vi "Funktionen Schalten Compact LP.vi"(8 "Fehler (Eingang)":errorcluster) -> (0 "Fehler (Ausgang)":errorcluster, 2 "Zustand":T1)   [LabVIEW 2020, in "Allgemein.lvlib"]
uses:
  Allgemein.lvlib
  Funktionstasten/Zustaende.ctl
  FGV Zustaende Aktionen.ctl
  Verwaltung/FGV OUT Aktionen.ctl
  Regler/FGV Daten Regler Aktionen.ctl
  Aktion FGV Messbetrieb.ctl
  Aktionen FGV Dichtheitstest.ctl
  Verwaltung/Verwaltung - cRIO.lvlib
  Regler/Regler.lvlib
  Funktionstasten/Funktionstasten.lvlib
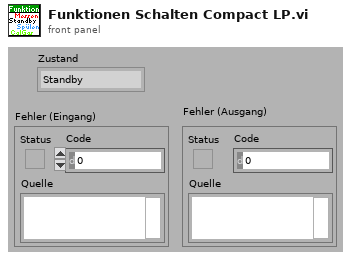
[diagram p1: front panel]
types:
  T1 = typedef "Funktionstasten.lvlib/Zustaende.ctl" = enum16{"Standby", "Pause", "Eco", "Messen", "Kalibrieren", "Spülen Filter", "Spülen Leitung", "Umgebungsluft", "0-Gas", "Cal-Gas", "CG zu PNS", "-------------", "Init 1", "Init 2", "Init 3", "Init 4", "Messen vorbereiten", "Messen durchführen", "Exit"}
  T2 = typedef "Allgemein.lvlib/Aktion FGV Messbetrieb.ctl" = enum16{"lesen", "schreiben"}
  T3 = typedef "Regler.lvlib/FGV Daten Regler Aktionen.ctl" = enum16{"lesen", "Out%", "Heizung EIN"}
  T4 = typedef "Verwaltung - cRIO.lvlib/FGV OUT Aktionen.ctl" = enum16{"lesen", "ANA OUT", "DO 0-31", "DO 32-47"}
  T5 = typedef "Allgemein.lvlib/FGV Zustaende Aktionen.ctl" = enum16{"lesen", "Zustand PC", "Zustand cRIO", "Bildnummer", "Samplepoint", "Sysloglevel"}
  T6 = typedef "Allgemein.lvlib/Aktionen FGV Dichtheitstest.ctl" = enum16{"lesen", "schreiben"}
  T7 = typedef "EPA 1065.lvlib/Dichtheitstest 1065-345.lvlib/Aktion Leak check durchfuehren.ctl" = enum16{"initialisieren", "Unterdruck erzeugen", "Ventile schließen", "Warten", "Auswertung", "fertig", "PDF erstellen", "abbrechen"}
  T8 = typedef "Erweiterte Konfig.lvlib/Aktionen Dichtheitstest.ctl" = enum16{"Initialisieren", "Unterdruck aufbauen", "Prop schließen", "Warten", "Auswertung", "Fertig"}
  T9 = cluster{"-23Y1":bool, "-23Y2":bool, "-23Y3":bool, "-23Y4":bool, "-23Y5":bool, "-27Y2":bool, "-20Y5":bool, "-20Y6":bool, "-20Y7":bool, "-20Y8":bool, "-27Y3":bool, "-27Y4":bool, "Pumpe":bool, "Kondensat":bool, "-22Y3":bool, "-20Y2":bool, "-21Y3":bool, "Absaugung":bool, "-21Y5":bool, "CG zu Entnahme":bool}
  T10 = cluster{"-23Y1 (Reserve)":bool, "-23Y2 (Reserve)":bool, "-23Y3 (CG1-8)":bool, "-23Y4 (N2)":bool, "-23Y5":bool, "-27Y2":bool, "-20Y5":bool, "-20Y6":bool, "-20Y7":bool, "-20Y8":bool, "-27Y3":bool, "-27Y4":bool, "Pumpe":bool, "Kondensat":bool, "-22Y3":bool, "-20Y2":bool, "-21Y3":bool, "Absaugung":bool, "-21Y5":bool, "CG zu Entnahme":bool, "-20Y2 (CG1)":bool, "-20Y3 (CG2)":bool, "-20Y4 (CG3)":bool, "-20Y5 (CG4)":bool, "-20Y6 (CG5)":bool, "-20Y7 (CG6)":bool, "-20Y8 (CG7)":bool, "-21Y1 (CG8)":bool}
  T11 = typedef "Verwaltung - cRIO.lvlib/Digital Ausgaenge 32-63.ctl" = cluster{"O32: Messgaspumpe EIN":bool, "O33: (Umgebungsluftpumpe)":bool, "O34: (Kondensatpumpe GK)":bool, "O35: Klima/Lüfter EIN":bool, "O36: Versorgung Heizungen":bool, "O37: Versorgung Heizungen":bool, "O38: (Gaskühler EIN (Freigabe))":bool, "O39: Störung FAS LP":bool, "O40: (Heizung Filterblock)":bool, "O41: Heizung HL zu FT-IR":bool, "O42: Heizung HL Extern SP1":bool, "O43: Heizung HL Extern SP2":bool, "O44: Heizung Reserve":bool, "O45: Heizung Reserve":bool, "O46: Statusbeleuchtung grün":bool, "O47: Statusbeleuchtung rot":bool}
  T12 = typedef "Verwaltung - cRIO.lvlib/Digital Ausgaenge 0-31.ctl" = cluster{"O0: Druckluft Versorgung":bool, "O1: CG 1 (FB Eingang 1)":bool, "O2: CG 2 (Kühlung FT-IR EIN)":bool, "O3: CG 3 (FB Bypass)":bool, "O4: CG 4 (FB CalGas)":bool, "O5: CG 5 (FB spülen/UL)":bool, "O6: CG 6 (FB zum FT-IR)":bool, "O7: CG 7 (FB zum FID)":bool, "O8: CG 8 (FB Reserve)":bool, "O9: (FB Reserve)":bool, "O10: (FB Umgebungsluft FID)":bool, "O11: (FB zum Gaskühler)":bool, "O12: FB Stickstoff zu FT-IR":bool, "O13: Optikbox FT-IR spülen":bool, "O14: (Purifier deaktivieren)":bool, "O15: (Umschaltung Purifier/Stickstoff)":bool, "O16: N2 Einblasung":bool, "O17: LSP LN2 Nachfüllung":bool, "O18: (Reserve)":bool, "O19: (Pumpe Eingang1)":bool, "O20: (Pumpe Eingang2)":bool, "O21: (Pumpe Spülen1)":bool, "O22: (Pumpe Spülen2)":bool, "O23: (Reserve)":bool, "O24: CalGas 1":bool, "O25: CalGas 2":bool, "O26: CG 3-8 (CalGas 3)":bool, "O27: Stickstoff aufschalten":bool, "O28: CG zu PNS":bool, "O29: FTIR Standby Spülung":bool, "O30: CG zu Entnahme(T90)":bool, "O31: (Purifier regenerieren)":bool}
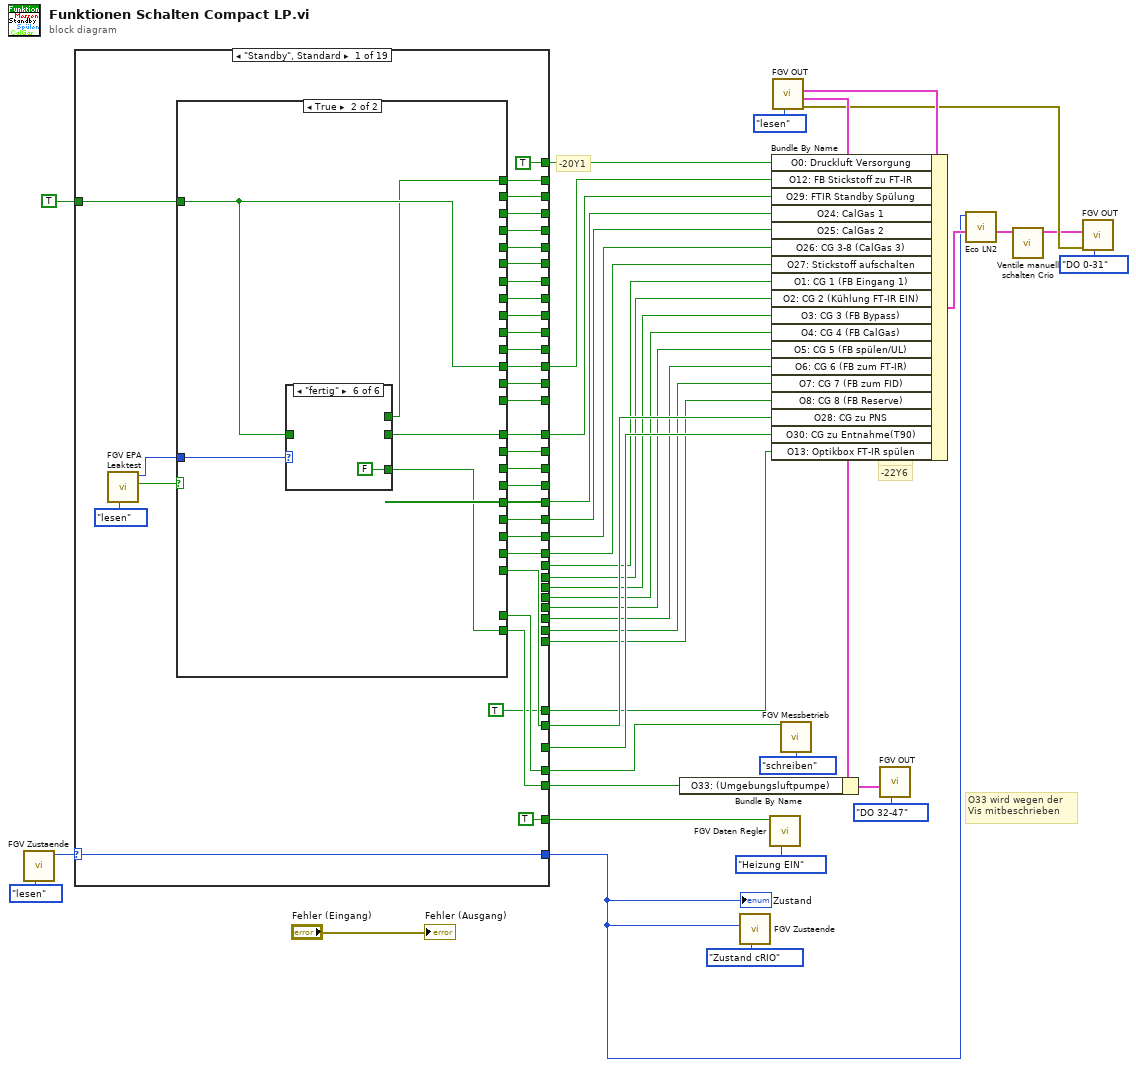
[diagram p0: block diagram]
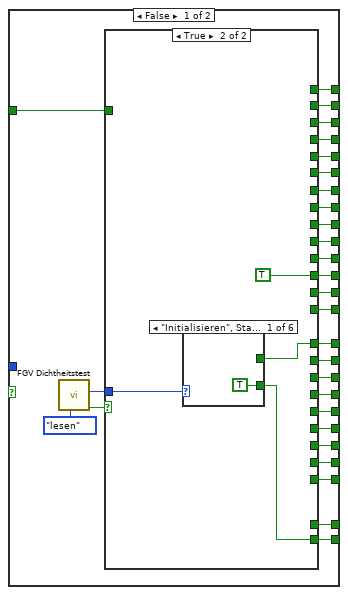
[diagram p2: hidden frame]
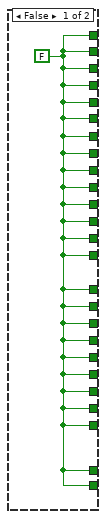
[diagram p3: hidden frame]
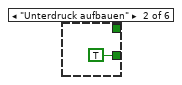
[diagram p4: hidden frame]
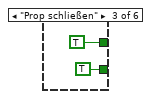
[diagram p5: hidden frame]
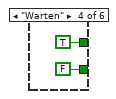
[diagram p6: hidden frame]
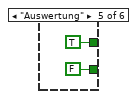
[diagram p7: hidden frame]
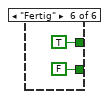
[diagram p8: hidden frame]
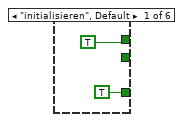
[diagram p9: hidden frame]
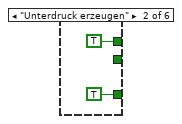
[diagram p10: hidden frame]
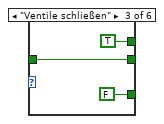
[diagram p11: hidden frame]
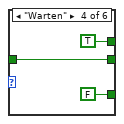
[diagram p12: hidden frame]
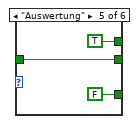
[diagram p13: hidden frame]
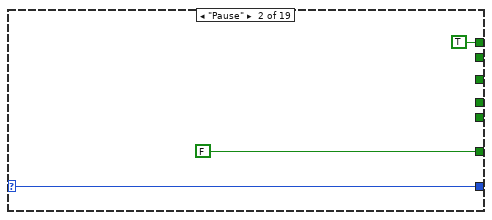
[diagram p14: hidden frame]
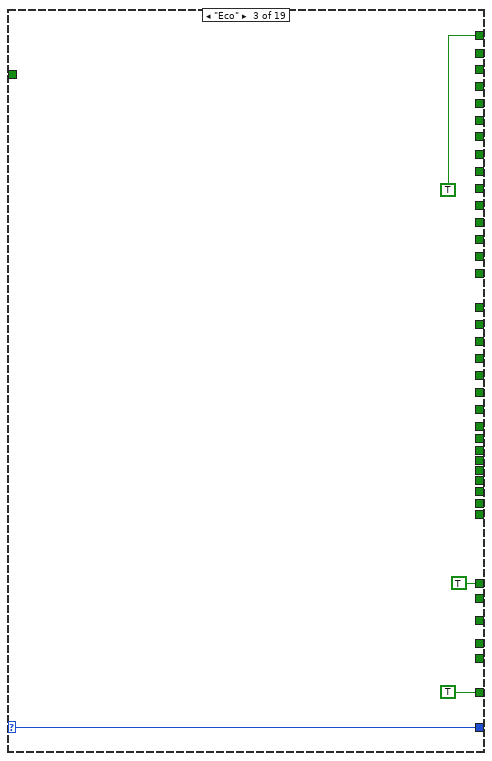
[diagram p15: hidden frame]
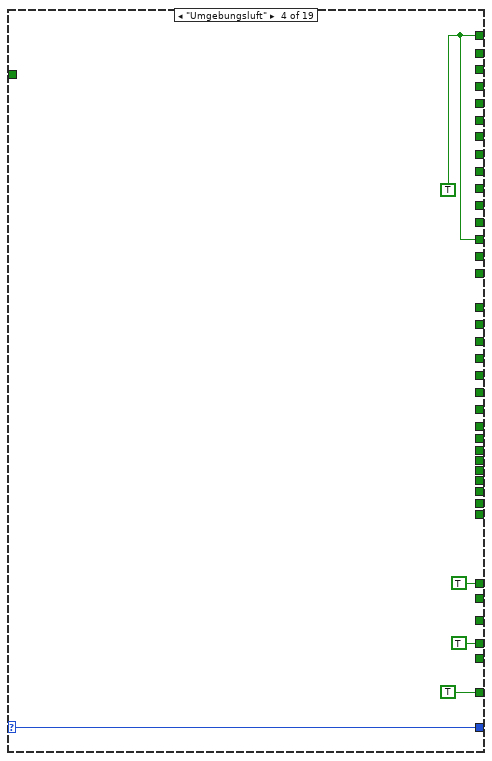
[diagram p16: hidden frame]
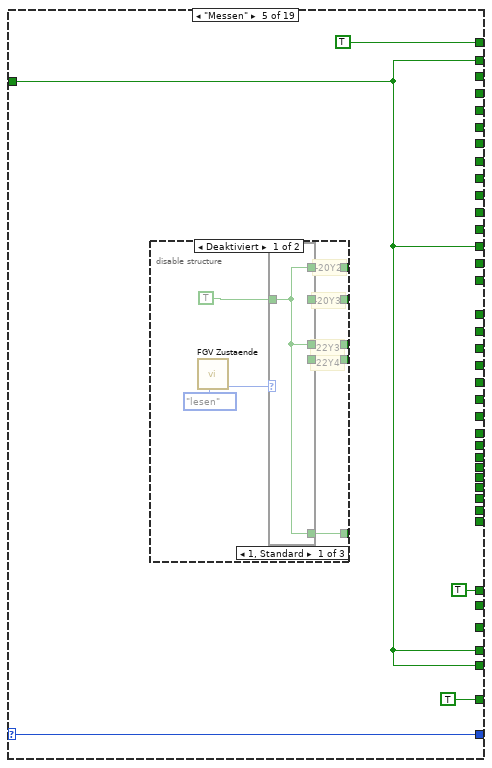
[diagram p17: hidden frame]
diagram:
  # "O33 wird wegen der \nVis mitbeschrieben"
  # "-20Y1"
  # "-22Y6"
  # "-22Y5"
  # "-22Y4"
  n1 = call "FGV Zustaende.vi"("Aktionen"=FGV_Zustaende_Aktionen."lesen") -> ("Zustand PC"=w31:T1)  [unwired: 6 in, 4 out]
  n2 = case shown="\"Standby\", Standard" w31 {
    selector: w31 -> [w72 w138 w142 w147 w152 w195 w219 w224 w241 w268 w331 _ _ _ _ _ w379 w381 _]
    tunnel: [w72 w138 w142 w147 w152 w195 w219 w224 w241 w268 w331 _ _ _ _ _ w379 w381 _] -> w14
    tunnel: [w70 _ _ _ w149 w189 _ w221 _ w265 w328 _ _ _ _ _ _ _ _] -> _
    tunnel: [w69 _ _ _ _ w188 _ _ _ _ _ _ _ _ _ _ _ _ _] -> _
    tunnel: [w67 _ _ _ _ w186 _ _ w238 w264 w327 _ _ _ _ _ _ _ _] -> _
    tunnel: [w66 _ _ _ _ w185 _ _ _ w263 w326 _ _ _ _ _ _ _ _] -> _
    tunnel: [w65 _ _ _ _ w184 _ _ _ w262 w325 _ _ _ _ _ _ _ _] -> _
    tunnel: [w64 _ _ _ _ w183 _ _ _ w261 w324 _ _ _ _ _ _ _ _] -> _
    tunnel: [w63 _ _ _ _ w181 _ _ _ _ _ _ _ _ _ _ _ _ _] -> _
    tunnel: [w61 _ _ w145 w149 w178 _ _ w239 w259 w323 _ _ _ _ _ _ _ _] -> w37
    tunnel: [w60 _ _ _ _ w177 w216 w221 _ _ _ _ _ _ _ _ _ _ _] -> _
    tunnel: TRUE -> [w71 _ _ _ w149 _ w216 w221 w239 _ _ _ _ _ _ _ _ _ _]
    tunnel: [w68 _ _ _ _ w187 w215 _ _ _ _ _ _ _ _ _ _ _ _] -> _
    tunnel: [w59 _ _ _ _ w176 _ _ _ _ _ _ _ _ _ _ _ _ _] -> _
    tunnel: [w51 _ _ _ w149 w166 _ _ w239 w242 w318 _ _ _ _ _ _ _ _] -> w21
    tunnel: [w52 _ _ TRUE ("Pumpe") w149 w165 _ _ TRUE ("Pumpe") TRUE ("Pumpe") w317 _ _ _ _ _ _ _ _] -> w18
    tunnel: [w54 _ _ _ _ w171 _ _ _ w258 w322 _ _ _ _ _ _ _ _] -> w4
    tunnel: [w55 _ _ _ _ w172 _ _ _ _ _ _ _ _ _ _ _ _ _] -> _
    tunnel: [w56 _ _ _ _ w173 _ _ _ _ _ _ _ _ _ _ _ _ _] -> _
    tunnel: [w57 _ _ _ _ w174 _ _ _ _ _ _ _ _ _ _ _ _ _] -> _
    tunnel: [w58 _ _ _ _ w175 _ _ _ _ _ _ _ _ _ _ _ _ _] -> w36
    tunnel: [w53 _ _ _ _ w169 _ _ _ w256 w320 _ _ _ _ _ _ _ _] -> w35
    tunnel: [TRUE ("O0: Druckluft Versorgung") _ TRUE ("O0: Druckluft Versorgung") w145 TRUE ("O0: Druckluft Versorgung") TRUE ("O0: Druckluft Versorgung") TRUE ("O0: Druckluft Versorgung") TRUE ("O0: Druckluft Versorgung") w238 TRUE ("O0: Druckluft Versorgung") TRUE ("O0: Druckluft Versorgung") _ _ _ _ _ _ _ _] -> w38
    tunnel: [w49 _ _ _ _ w182 _ _ _ _ _ _ _ _ _ _ _ _ _] -> _
    tunnel: [w48 _ _ _ _ w179 _ _ _ _ _ _ _ _ _ _ _ _ _] -> _
    tunnel: [w47 _ _ _ _ w170 _ _ _ w257 w321 _ _ _ _ _ _ _ _] -> w3
    tunnel: [w46 _ _ _ _ w167 _ _ _ w252 w316 _ _ _ _ _ _ _ _] -> w34
    tunnel: [w45 _ _ _ _ w168 _ _ w239 w255 w319 _ _ _ _ _ _ _ _] -> w33
    tunnel: [TRUE ("Heizung AUS") FALSE ("Heizung AUS") TRUE ("Heizung AUS") TRUE ("Heizung AUS") TRUE ("Heizung AUS") TRUE ("Heizung AUS") TRUE ("Heizung AUS") TRUE ("Heizung AUS") TRUE ("Heizung AUS") TRUE ("Heizung AUS") TRUE ("Heizung AUS") TRUE ("Heizung AUS") _ _ _ _ _ _ _] -> w22
    tunnel: [w62 _ _ _ _ w180 _ _ _ w260 w315 _ _ _ _ _ _ _ _] -> _
    tunnel: [_ _ _ _ _ _ _ _ _ w253 w314 _ _ _ _ _ _ _ _] -> w17
    tunnel: [_ _ _ _ _ _ _ _ _ w251 w313 _ _ _ _ _ _ _ _] -> w13
    tunnel: [_ _ _ _ _ _ _ _ _ w250 w312 _ _ _ _ _ _ _ _] -> w12
    tunnel: [_ _ _ _ _ _ _ _ _ w249 w311 _ _ _ _ _ _ _ _] -> w11
    tunnel: [_ _ _ _ _ _ _ _ _ w248 w310 _ _ _ _ _ _ _ _] -> w10
    tunnel: [_ _ _ _ _ _ _ _ _ w247 w309 _ _ _ _ _ _ _ _] -> w9
    tunnel: [_ _ _ _ _ _ _ _ _ w246 w308 _ _ _ _ _ _ _ _] -> w8
    tunnel: [_ _ _ _ _ _ _ _ _ w245 w307 _ _ _ _ _ _ _ _] -> w7
    tunnel: [_ _ _ _ _ _ _ _ _ w244 w306 _ _ _ _ _ _ _ _] -> w6
    tunnel: [TRUE ("Heizung AUS") TRUE ("Heizung AUS") TRUE ("Heizung AUS") TRUE ("Heizung AUS") TRUE ("Heizung AUS") TRUE ("Heizung AUS") TRUE ("Heizung AUS") TRUE ("Heizung AUS") TRUE ("Heizung AUS") TRUE ("Heizung AUS") TRUE ("Heizung AUS") TRUE ("Heizung AUS") TRUE ("Heizung AUS") TRUE ("Heizung AUS") TRUE ("Heizung AUS") TRUE ("Heizung AUS") TRUE ("Heizung AUS") TRUE ("Heizung AUS") TRUE ("Heizung AUS")] -> w5
    frame "Standby", Default {
      n3 = call "FGV EPA Leaktest.vi"("Aktion"=enum16{"lesen", "schreiben"}."lesen") -> ("Leaktest aktiv"=w42:bool, "Leaktest Zustand"=w41:T7)  [unwired: 9 in]
      n4 = case shown="True" w42 {
        tunnel: w71 -> [w101 w119]
        tunnel: [w100 w118] -> w70
        tunnel: [w99 _] -> w69
        tunnel: [w98 _] -> w68
        tunnel: [w97 _] -> w67
        tunnel: [w96 _] -> w66
        tunnel: [w95 _] -> w65
        tunnel: [w94 _] -> w64
        tunnel: [w93 _] -> w63
        tunnel: [w92 _] -> w62
        tunnel: [w91 w119] -> w61
        tunnel: [w90 _] -> w60
        tunnel: [w89 _] -> w59
        tunnel: [w88 w120] -> w58
        tunnel: [w87 _] -> w57
        tunnel: [w86 _] -> w56
        tunnel: [w85 _] -> w55
        tunnel: [w84 _] -> w54
        tunnel: [w83 _] -> w53
        tunnel: [w82 _] -> w52
        tunnel: [w81 w117] -> w51
        tunnel: [w78 _] -> w49
        tunnel: [w77 _] -> w48
        tunnel: [w76 _] -> w47
        tunnel: [w75 _] -> w46
        tunnel: [w74 _] -> w45
        tunnel: w41 -> [_ w121]
        frame False {
          n5 = call "FGV Dichtheitstest.vi"("Aktionen"=Aktionen_FGV_Dichtheitstest."lesen") -> ("Dichtheitstest?"=w79:bool, "Aktionen Dichtheitstest"=w73:T8)  [unwired: 9 in]
          n6 = case shown="True" w79 {
            tunnel: [w102 _] -> w100
            tunnel: [w102 w103] -> w81
            tunnel: [w102 _] -> w82
            tunnel: [w102 _] -> w83
            tunnel: [w102 _] -> w84
            tunnel: [w102 _] -> w85
            tunnel: [w102 _] -> w86
            tunnel: [w102 _] -> w87
            tunnel: [w102 w104] -> w88
            tunnel: [w102 _] -> w89
            tunnel: [w102 _] -> w90
            tunnel: [w102 TRUE] -> w91
            tunnel: [w102 _] -> w92
            tunnel: [w102 _] -> w93
            tunnel: [w102 _] -> w94
            tunnel: [w102 _] -> w95
            tunnel: [w102 _] -> w96
            tunnel: [w102 _] -> w97
            tunnel: [w102 _] -> w98
            tunnel: [w102 _] -> w99
            tunnel: w101 -> [_ _]
            tunnel: [w102 _] -> w78
            tunnel: [w102 _] -> w77
            tunnel: [w102 _] -> w76
            tunnel: [w102 _] -> w75
            tunnel: [w102 _] -> w74
            tunnel: w73 -> [_ w105]
            frame False {
              w102 = FALSE
            }
            frame True {
              n7 = case shown="\"Initialisieren\", Standard" w105 {
                tunnel: [_ _ TRUE TRUE TRUE TRUE] -> w104
                tunnel: [TRUE TRUE TRUE FALSE FALSE FALSE] -> w103
                frame "Initialisieren", Default {
                }
                frame "Unterdruck aufbauen" {
                }
                frame "Prop schließen" {
                }
                frame "Warten" {
                }
                frame "Auswertung" {
                }
                frame "Fertig" {
                }
              }
            }
          }
        }
        frame True {
          n8 = case shown="\"fertig\"" w121 {
            tunnel: w119 -> [_ _ w128 w131 w134 _]
            tunnel: [_ _ w128 w131 w134 _] -> w120
            tunnel: [TRUE TRUE TRUE TRUE TRUE _] -> w118
            tunnel: [TRUE TRUE FALSE FALSE FALSE FALSE] -> w117
            frame "initialisieren", Default {
            }
            frame "Unterdruck erzeugen" {
            }
            frame "Ventile schließen" {
            }
            frame "Warten" {
            }
            frame "Auswertung" {
            }
            frame "fertig" {
            }
          }
        }
      }
    }
    frame "Pause" {
    }
    frame "Eco" {
    }
    frame "Umgebungsluft" {
      w145 = TRUE ("O0: Druckluft Versorgung")
    }
    frame "Messen" {
      n9 = disable-structure shown="Deaktiviert" {
        disable-tunnel: [w160 _] -> _
        disable-tunnel: [w159 _] -> _
        disable-tunnel: [w158 _] -> _
        disable-tunnel: [w157 _] -> _
        disable-tunnel: [w156 _] -> _
        frame Disabled {
          # "-22Y4"
          # "-22Y3"
          # "-20Y2"
          # "-20Y3"
          n10 = call "FGV Zustaende.vi"("Aktionen"=FGV_Zustaende_Aktionen."lesen") -> ("Samplepoint"=w153:u16)  [unwired: 6 in, 4 out]
          n11 = case shown="1, Standard" w153 {
            tunnel: TRUE -> [w161 w162 w163]
            tunnel: [w161 _ _] -> w160
            tunnel: [w161 w162 _] -> w159
            tunnel: [_ w162 _] -> w158
            tunnel: [_ _ w163] -> w157
            tunnel: [w161 w162 _] -> w156
            frame 1, Default {
            }
            frame 2 {
            }
            frame 3 {
            }
          }
        }
        frame Enabled {
        }
      }
    }
    frame "Kalibrieren" {
      n12 = call "FGV Dichtheitstest.vi"("Aktionen"=Aktionen_FGV_Dichtheitstest."lesen") -> ("Dichtheitstest?"=w191:bool, "Aktionen Dichtheitstest"=w190:T8)  [unwired: 9 in]
      n13 = case shown="False" w191 {
        tunnel: [w198 _] -> w189
        tunnel: [w198 w199] -> w166
        tunnel: [w197 _] -> w165
        tunnel: [w198 _] -> w169
        tunnel: [w198 _] -> w171
        tunnel: [w198 _] -> w172
        tunnel: [w198 _] -> w173
        tunnel: [w198 _] -> w174
        tunnel: [w198 w200] -> w175
        tunnel: [w198 _] -> w176
        tunnel: [w198 _] -> w177
        tunnel: [TRUE TRUE] -> w178
        tunnel: [w198 _] -> w180
        tunnel: [w198 _] -> w181
        tunnel: [w198 _] -> w183
        tunnel: [w198 _] -> w184
        tunnel: [w198 _] -> w185
        tunnel: [w198 _] -> w186
        tunnel: [w198 _] -> w187
        tunnel: [w198 _] -> w188
        tunnel: [w198 _] -> w182
        tunnel: [w198 _] -> w179
        tunnel: [w198 _] -> w170
        tunnel: [w197 _] -> w167
        tunnel: [w197 _] -> w168
        tunnel: w190 -> [_ w201]
        frame False {
          w197 = TRUE
          w198 = FALSE
        }
        frame True {
          n14 = case shown="\"Warten\"" w201 {
            tunnel: [_ _ TRUE TRUE TRUE TRUE] -> w200
            tunnel: [TRUE TRUE TRUE FALSE FALSE FALSE] -> w199
            frame "Initialisieren", Default {
            }
            frame "Unterdruck aufbauen" {
            }
            frame "Prop schließen" {
            }
            frame "Warten" {
            }
            frame "Auswertung" {
            }
            frame "Fertig" {
            }
          }
        }
      }
    }
    frame "Spülen Filter" {
      n15 = call "Taktmerker.vi"("Aktion"=enum16{"lesen", "bearbeiten"}."lesen") -> ("1 s"=w215:bool)  [unwired: 6 in, 4 out]
    }
    frame "Spülen Leitung" {
      n16 = disable-structure shown="Deaktiviert" {
        disable-tunnel: [w232 _] -> _
        disable-tunnel: [w231 _] -> _
        disable-tunnel: [w230 _] -> _
        disable-tunnel: [w229 _] -> _
        disable-tunnel: [w228 _] -> _
        frame Disabled {
          # "-22Y6"
          # "-22Y5"
          # "-21Y7"
          # "-20Y6"
          # "-20Y3"
          n17 = call "FGV Zustaende.vi"("Aktionen"=FGV_Zustaende_Aktionen."lesen") -> ("Samplepoint"=w225:u16)  [unwired: 6 in, 4 out]
          n18 = case shown="3" w225 {
            tunnel: TRUE -> [w233 w234 w235]
            tunnel: [w233 _ _] -> w232
            tunnel: [_ w234 _] -> w231
            tunnel: [_ _ w235] -> w230
            tunnel: [_ _ w235] -> w229
            tunnel: [_ _ w235] -> w228
            frame 1, Default {
            }
            frame 2 {
            }
            frame 3 {
            }
          }
        }
        frame Enabled {
        }
      }
    }
    frame "0-Gas" {
      w238 = TRUE ("O0: Druckluft Versorgung")
    }
    frame "Cal-Gas" {
      n19 = disable-structure shown="Paccar==TRUE" {
        disable-tunnel: [w282 w303] -> w265
        disable-tunnel: [w281 w302] -> w264
        disable-tunnel: [w280 w301] -> w263
        disable-tunnel: [w279 w300] -> w262
        disable-tunnel: [w278 w299] -> w261
        disable-tunnel: [w277 w298] -> w260
        disable-tunnel: [w276 w297] -> w259
        disable-tunnel: [w275 _] -> w258
        disable-tunnel: [w274 _] -> w257
        disable-tunnel: [w273 w296] -> w256
        disable-tunnel: [w272 w295] -> w255
        disable-tunnel: [w271 w294] -> w242
        disable-tunnel: [w270 w293] -> w253
        disable-tunnel: [w269 w292] -> w252
        disable-tunnel: [_ w291] -> w251
        disable-tunnel: [_ w290] -> w250
        disable-tunnel: [_ w289] -> w249
        disable-tunnel: [_ w288] -> w248
        disable-tunnel: [_ w287] -> w247
        disable-tunnel: [_ w286] -> w246
        disable-tunnel: [_ w285] -> w245
        disable-tunnel: [_ w284] -> w244
        frame condition #0 (active) {
          n20 = call "CalGas aufschalten.vi"() -> ("Cluster"=w283:T9)  [unwired: 11 in]
          n21 = Unbundle By Name(w283) -> ("-20Y2"=w282:bool, "-20Y5"=w281:bool, "-20Y6"=w280:bool, "-20Y7"=w279:bool, "-20Y8"=w278:bool, "-21Y3"=w277:bool, "-21Y5"=w276:bool, "-23Y1"=w275:bool, "-23Y2"=w274:bool, "-23Y3"=w273:bool, "-23Y4"=w272:bool, "-23Y5"=w269:bool, "Absaugung"=w271:bool, "CG zu Entnahme"=w270:bool)  [unwired: 5 out]
        }
        frame condition #1 {
          n22 = call "CalGas aufschalten Paccar.vi"() -> ("Cluster"=w304:T10)  [unwired: 11 in]
          n23 = Unbundle By Name(w304) -> ("-20Y2"=w303:bool, "-20Y5"=w302:bool, "-20Y6"=w301:bool, "-20Y7"=w300:bool, "-20Y8"=w299:bool, "-21Y3"=w298:bool, "-21Y5"=w297:bool, "-23Y3 (CG1-8)"=w296:bool, "-23Y4 (N2)"=w295:bool, "-20Y2 (CG1)"=w291:bool, "-20Y3 (CG2)"=w290:bool, "-20Y4 (CG3)"=w289:bool, "-20Y5 (CG4)"=w288:bool, "-20Y6 (CG5)"=w287:bool, "-20Y7 (CG6)"=w286:bool, "-20Y8 (CG7)"=w285:bool, "-21Y1 (CG8)"=w284:bool, "-23Y5"=w292:bool, "Absaugung"=w294:bool, "CG zu Entnahme"=w293:bool)  [unwired: 2 out]
        }
      }
    }
    frame "CG zu PNS" {
      n24 = disable-structure shown="AK_Paccar==TRUE" {
        disable-tunnel: [w346 w371] -> w328
        disable-tunnel: [w345 w370] -> w327
        disable-tunnel: [w344 w369] -> w326
        disable-tunnel: [w343 w368] -> w325
        disable-tunnel: [w342 w367] -> w324
        disable-tunnel: [w341 w366] -> w323
        disable-tunnel: [w340 w365] -> w322
        disable-tunnel: [w339 w364] -> w321
        disable-tunnel: [w338 w363] -> w320
        disable-tunnel: [w337 w362] -> w319
        disable-tunnel: [w336 w361] -> w318
        disable-tunnel: [w335 w360] -> w317
        disable-tunnel: [w334 w359] -> w316
        disable-tunnel: [w333 w358] -> w315
        disable-tunnel: [w332 w357] -> w314
        disable-tunnel: [_ w355] -> w313
        disable-tunnel: [_ w354] -> w312
        disable-tunnel: [_ w353] -> w311
        disable-tunnel: [_ w352] -> w310
        disable-tunnel: [_ w351] -> w309
        disable-tunnel: [_ w350] -> w308
        disable-tunnel: [_ w349] -> w307
        disable-tunnel: [_ w348] -> w306
        frame condition #0 (active) {
          n25 = call "CalGas aufschalten.vi"() -> ("Cluster"=w347:T9)  [unwired: 11 in]
          n26 = Unbundle By Name(w347) -> ("-20Y2"=w346:bool, "-20Y5"=w345:bool, "-20Y6"=w344:bool, "-20Y7"=w343:bool, "-20Y8"=w342:bool, "-21Y3"=w333:bool, "-21Y5"=w341:bool, "-23Y1"=w340:bool, "-23Y2"=w339:bool, "-23Y3"=w338:bool, "-23Y4"=w337:bool, "-23Y5"=w334:bool, "Pumpe"=w335:bool, "Absaugung"=w336:bool, "CG zu Entnahme"=w332:bool)  [unwired: 4 out]
        }
        frame condition #1 {
          n27 = call "CalGas aufschalten Paccar.vi"() -> ("Cluster"=w356:T10)  [unwired: 11 in]
          n28 = Unbundle By Name(w356) -> ("-20Y2"=w371:bool, "-20Y5"=w370:bool, "-20Y6"=w369:bool, "-20Y7"=w368:bool, "-20Y8"=w367:bool, "-21Y3"=w358:bool, "-21Y5"=w366:bool, "-23Y1 (Reserve)"=w365:bool, "-23Y2 (Reserve)"=w364:bool, "-23Y3 (CG1-8)"=w363:bool, "-23Y4 (N2)"=w362:bool, "-23Y5"=w359:bool, "Pumpe"=w360:bool, "Absaugung"=w361:bool, "CG zu Entnahme"=w357:bool, "-20Y2 (CG1)"=w355:bool, "-20Y3 (CG2)"=w354:bool, "-20Y4 (CG3)"=w353:bool, "-20Y5 (CG4)"=w352:bool, "-20Y6 (CG5)"=w351:bool, "-20Y7 (CG6)"=w350:bool, "-20Y8 (CG7)"=w349:bool, "-21Y1 (CG8)"=w348:bool)  [unwired: 4 out]
        }
      }
    }
    frame "-------------" {
    }
    frame "Init 1" {
    }
    frame "Init 2" {
    }
    frame "Init 3" {
    }
    frame "Init 4" {
    }
    frame "Messen vorbereiten" {
    }
    frame "Messen durchführen" {
    }
    frame "Exit" {
    }
  }
  "Zustand" <- w14
  n29 = call "FGV Zustaende.vi"("Aktionen"=FGV_Zustaende_Aktionen."Zustand cRIO", "Zustand cRIO"=w14) -> ()  [unwired: 5 in, 5 out]
  n30 = call "FGV Daten Regler.vi"("Aktionen"=FGV_Daten_Regler_Aktionen."Heizung EIN", "Heizung EIN"=w22) -> ()  [unwired: 8 in, 2 out]
  n31 = call "FGV OUT.vi"("Aktion"=FGV_OUT_Aktionen."lesen") -> ("error out"=w15:errorcluster, "DO 32-63"=w27:T11, "DO 0-31"=w28:T12)  [unwired: 7 in, 1 out]
  n32 = Bundle By Name(cluster=w27, "O33: (Umgebungsluftpumpe)"=w21) -> (w24:T11)
  n33 = Bundle By Name(cluster=w28, "O0: Druckluft Versorgung"=w38, "O12: FB Stickstoff zu FT-IR"=w37, "O29: FTIR Standby Spülung"=w36, "O24: CalGas 1"=w4, "O25: CalGas 2"=w3, "O26: CG 3-8 (CalGas 3)"=w35, "O27: Stickstoff aufschalten"=w33, "O1: CG 1 (FB Eingang 1)"=w13, "O2: CG 2 (Kühlung FT-IR EIN)"=w12, "O3: CG 3 (FB Bypass)"=w11, "O4: CG 4 (FB CalGas)"=w10, "O5: CG 5 (FB spülen/UL)"=w9, "O6: CG 6 (FB zum FT-IR)"=w8, "O7: CG 7 (FB zum FID)"=w7, "O8: CG 8 (FB Reserve)"=w6, "O28: CG zu PNS"=w34, "O30: CG zu Entnahme(T90)"=w17, "O13: Optikbox FT-IR spülen"=w5) -> (w16:T12)
  n34 = call "FGV Messbetrieb.vi"("messen"=w18, "Aktion"=Aktion_FGV_Messbetrieb."schreiben") -> ()  [unwired: 12 in, 2 out]
  n35 = call "FGV OUT.vi"("Aktion"=FGV_OUT_Aktionen."DO 32-47", "DO 32-63"=w24) -> ()  [unwired: 6 in, 4 out]
  n36 = call "Eco LN2.vi"("DO 0-31"=w16, "Zustand cRIO"=w14) -> ("DO 0-31"=w2:T12)  [unwired: 8 in, 1 out]
  n37 = call "Ventile manuell schalten Crio.vi"("DO 0-31"=w2) -> ("DO 0-31"=w1:T12)  [unwired: 9 in, 1 out]
  n38 = call "FGV OUT.vi"("Aktion"=FGV_OUT_Aktionen."DO 0-31", "error in (no error)"=w15, "DO 0-31"=w1) -> ()  [unwired: 5 in, 4 out]
  "Fehler (Ausgang)" <- "Fehler (Eingang)"
